vi "Measurement Logic.vi"() -> ()   [LabVIEW 2021, in "Eff And Load Reg_Channel Ganging.lvlib"]
uses:
  Eff And Load Reg_Channel Ganging.lvlib
  Measurement Configuration.ctl
  Measurement Results.ctl
  <vilib>/Plug-In SDKs/Measurements/Measure Call Context/Measure Call Context.lvclass
  shared/Ganging/controls/Power ON-Ganging.ctl
  shared/Single/controls/Power ON-Single.ctl
panel:
  out "measure call context out":refnum<class "Measure Call Context.lvclass">
  in  "measure call context in":refnum<class "Measure Call Context.lvclass">
  out "measurement results":T1
  in  "measurement configuration":T2={"Mode of operation"=enum."Power on the DUT", "Source resource names"=[], "Load resource names"=[], "Power ON output function"=1006, "Power ON/Source system configuration"=enum."Parallel", "Power ON V/I Source start level"=6.0, "Source stop voltage"=14.0, "Source voltage sweep points"=4, "Source voltage level range"=20.0, "Power ON/Source sense"=1009, "Source limit symmetry"=enum."Asymmetric", "Power ON/Source current/voltage limit range"=25.0, "Source current limit low"=-0.6, "Source current limit high"=25.0, "Source transient response"=1038, "Source voltage gain bandwidth"=2000.0, "Source voltage compensation frequency"=3530.0, "Source voltage pole-zero ratio"=2.0, "Load system configuration"=enum."Parallel", "Load device voltage/current rating"=50.0, "Load start current"=1.0, "Load stop current"=50.0, "Load current sweep points/points per decade"=10, "Load sweep type"="Logarithmic", "Load current level range"=80.0, "Load sense"=1009, "Load limit symmetry"=enum."Symmetric", "Load voltage limit range"=6.0, "Load voltage limit low"=0.0, "Load voltage limit high"=inf, "Load transient response"=1038, "Load current gain bandwidth"=14000.0, "Load current compensation frequency"=180000.0, "Load current pole-zero ratio"=0.3, "DUT setup time"=1.0, "Source delay"=0.005, "Aperture time"=0.005, "Nominal output voltage"=1.0, "Measurement timeout"=10.0} {"Power ON output function" items=["Series", "Parallel", "Manual"]; "Nominal output voltage" format="%#_6pA"; "Source voltage sweep points" format="%#_6p"; "Power ON V/I Source start level" format="%#_6p"; "Load sense" items=["Symmetric", "Asymmetric"]; "Load transient response" items=["Slow"=1041, "Normal"=1038, "Fast"=1039, "Custom"=1042]; "Power ON/Source sense" items=["Symmetric", "Asymmetric"]; "Source transient response" items=["Slow"=1041, "Normal"=1038, "Fast"=1039, "Custom"=1042]; "Load voltage limit high" format="%#_6p"; "Load voltage limit low" format="%#_6p"; "Load voltage limit range" format="%#_6p"; "Load current level range" format="%#_6p"; "Source current limit high" format="%#_6p"; "Source current limit low" format="%#_6p"; "Power ON/Source current/voltage limit range" format="%#_6p"; "Source voltage level range" format="%#_6p"}
  out "error out":errorcluster
  in  "error in":errorcluster
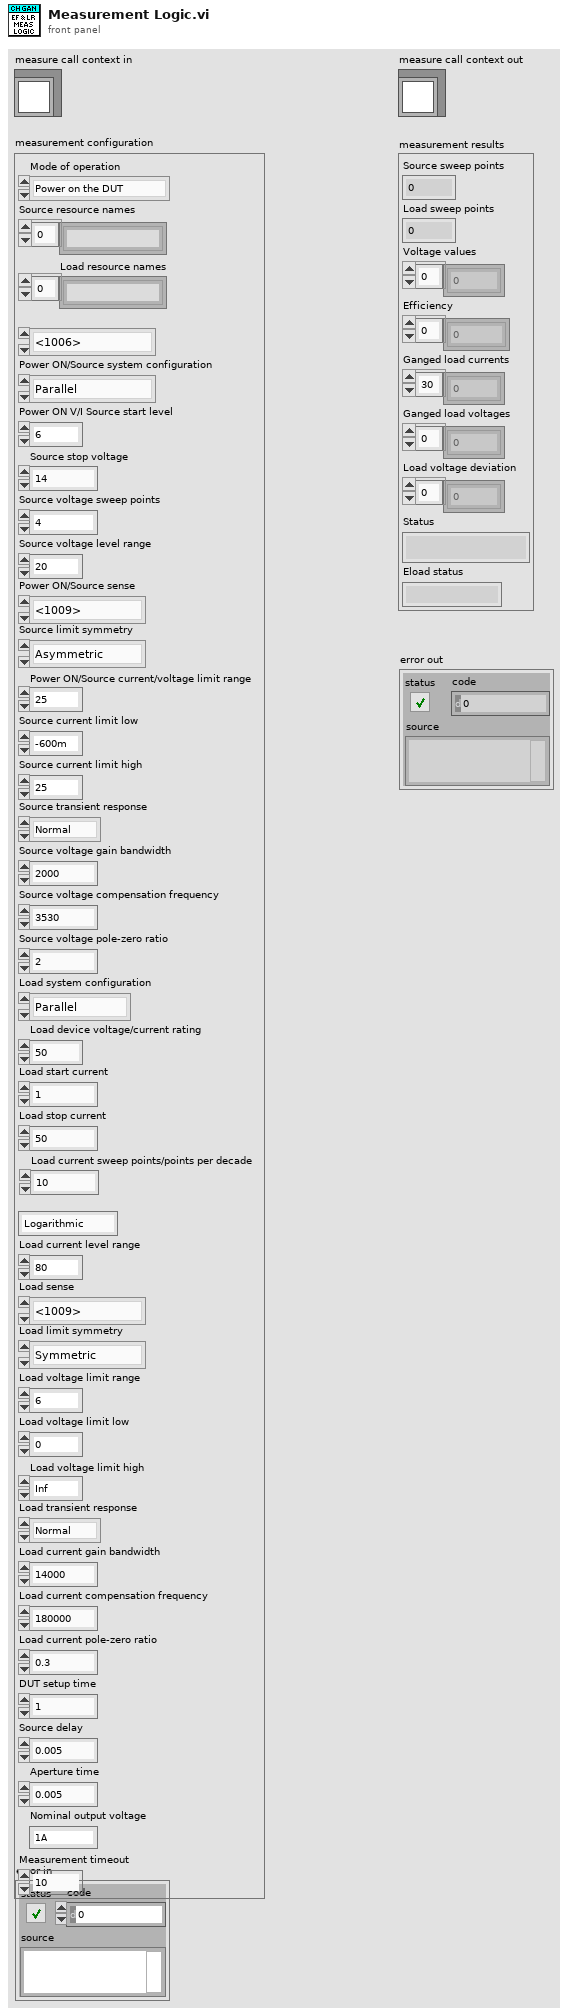
[diagram p1: front panel]
types:
  T1 = typedef "Eff And Load Reg_Channel Ganging.lvlib/Measurement Results.ctl" = cluster{"Source sweep points":i32, "Load sweep points":i32, "Voltage values":dbl[], "Efficiency":dbl[], "Ganged load currents":dbl[], "Ganged load voltages":dbl[], "Load voltage deviation":dbl[], "Status":string, "Eload status":string}
  T2 = typedef "Eff And Load Reg_Channel Ganging.lvlib/Measurement Configuration.ctl" = cluster{"Mode of operation":enum32{"Power on the DUT", "Perform measurement", "Power off the DUT"}, "Source resource names":string[], "Load resource names":string[], "Power ON output function":i32, "Power ON/Source system configuration":enum32{"Series", "Parallel", "Manual"}, "Power ON V/I Source start level":dbl, "Source stop voltage":dbl, "Source voltage sweep points":i32, "Source voltage level range":dbl, "Power ON/Source sense":i32, "Source limit symmetry":enum32{"Symmetric", "Asymmetric"}, "Power ON/Source current/voltage limit range":dbl, "Source current limit low":dbl, "Source current limit high":dbl, "Source transient response":i32, "Source voltage gain bandwidth":dbl, "Source voltage compensation frequency":dbl, "Source voltage pole-zero ratio":dbl, "Load system configuration":enum32{"Series", "Parallel", "Manual"}, "Load device voltage/current rating":dbl, "Load start current":dbl, "Load stop current":dbl, "Load current sweep points/points per decade":i32, "Load sweep type":string, "Load current level range":dbl, "Load sense":i32, "Load limit symmetry":enum32{"Symmetric", "Asymmetric"}, "Load voltage limit range":dbl, "Load voltage limit low":dbl, "Load voltage limit high":dbl, "Load transient response":i32, "Load current gain bandwidth":dbl, "Load current compensation frequency":dbl, "Load current pole-zero ratio":dbl, "DUT setup time":dbl, "Source delay":dbl, "Aperture time":dbl, "Nominal output voltage":dbl, "Measurement timeout":dbl}
  T3 = enum32{"Power on the DUT", "Perform measurement", "Power off the DUT"}
  T4 = typedef "Power ON-Ganging.ctl" = cluster{"Master/single Resource name":string, "Slave resource name":string[], "System configuration":enum32{"Series", "Parallel", "Manual"}, "Output function":i32, "Voltage/current level":dbl, "Voltage/current limit":dbl, "Sense":i32}
  T5 = typedef "Power ON-Single.ctl" = cluster{"Voltage/current level":dbl, "Voltage/current limit":dbl, "Sense":i32, "Resource name":string, "Output function":i32}
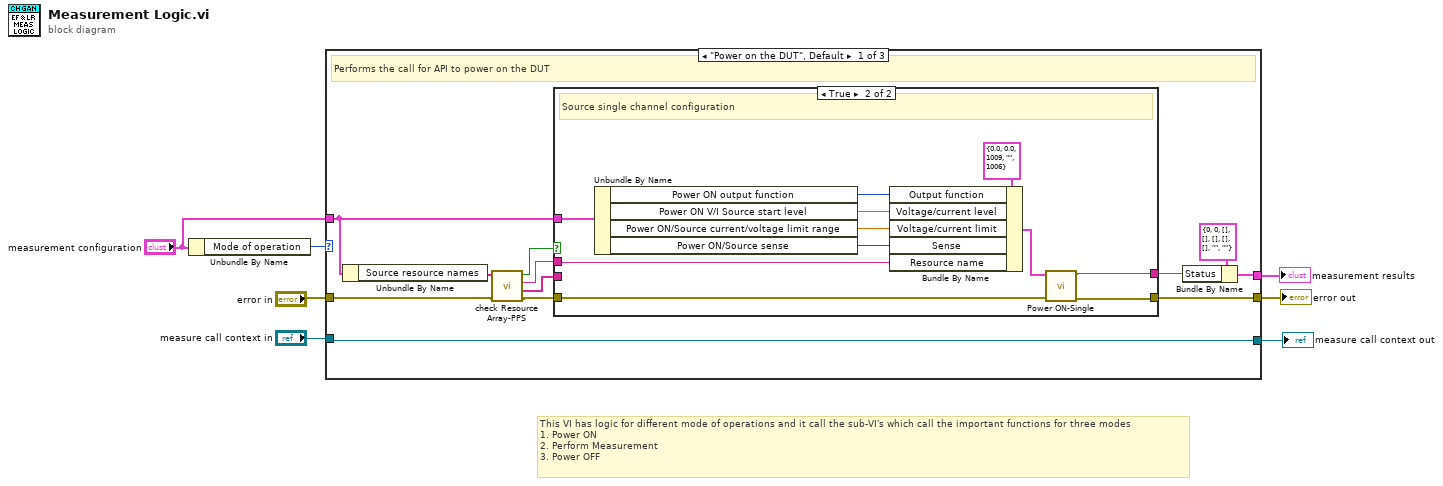
[diagram p0: block diagram]
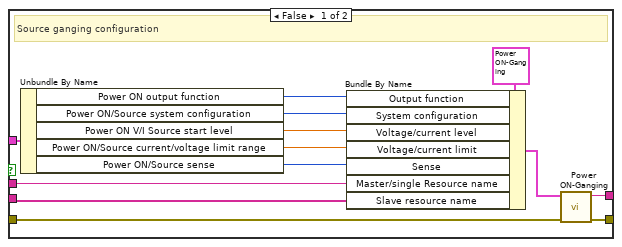
[diagram p2: hidden frame]
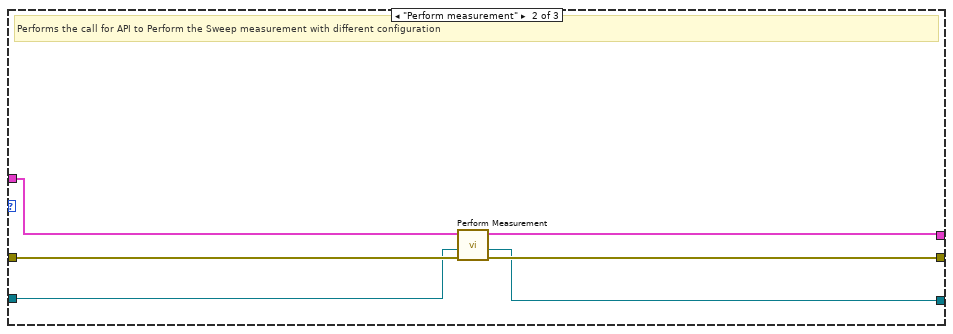
[diagram p3: hidden frame]
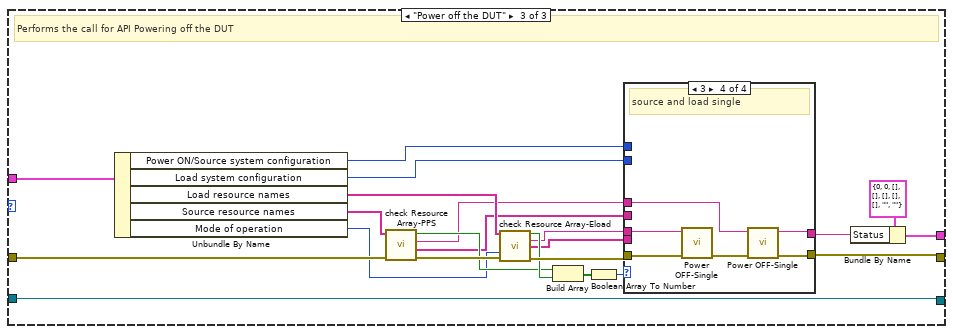
[diagram p4: hidden frame]
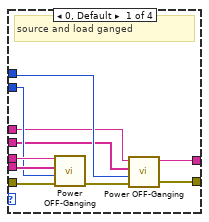
[diagram p5: hidden frame]
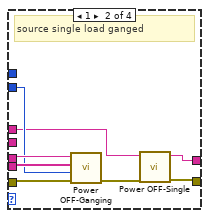
[diagram p6: hidden frame]
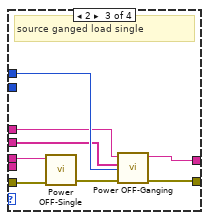
[diagram p7: hidden frame]
diagram:
  # "This VI has logic for different mode of operations and it call the sub-VI's which call the important functions for three modes\n1. Power ON\n2. Perform Measurement\n3. Power OFF"
  n1 = Unbundle By Name("measurement configuration") -> ("Mode of operation"=w7:T3)
  n2 = case shown="\"Power on the DUT\", Default" w7 {
    tunnel: "measurement configuration" -> [w14 w45 w57]
    tunnel: "error in" -> [w13 w49 w56]
    tunnel: [w12 w48 w55] -> w5
    tunnel: [w11 w47 w53] -> w3
    tunnel: "measure call context in" -> [w11 w46 w53]
    tunnel: [w8 w44 w51] -> w1
    frame "Power on the DUT", Default {
      # "Performs the call for API to power on the DUT"
      n3 = Unbundle By Name(w14) -> ("Source resource names"=w16:string[])
      n4 = call "check Resource Array-PPS.vi"("error in"=w13, "Resource names"=w16) -> ("error out"=w19:errorcluster, "Slave resource names"=w17:string[], "Single/Master resouce names"=w18:string, "Single or ganged configuration"=w15:bool)  [unwired: 6 in]
      n5 = case shown="True" w15 {
        tunnel: w19 -> [w27 w42]
        tunnel: [w28 w41] -> w12
        tunnel: w17 -> [w30 _]
        tunnel: w14 -> [w32 w43]
        tunnel: w18 -> [w31 w38]
        tunnel: [w29 w40] -> w10
        frame False {
          # "Source ganging configuration"
          n6 = Unbundle By Name(w32) -> ("Power ON output function"=w20:i32, "Power ON/Source system configuration"=w24:enum32{"Series", "Parallel", "Manual"}, "Power ON V/I Source start level"=w23:dbl, "Power ON/Source current/voltage limit range"=w22:dbl, "Power ON/Source sense"=w21:i32)
          n7 = Bundle By Name(cluster=T4 {"Master/single Resource name"="", "Slave resource name"=[], "System configuration"=enum."Parallel", "Output function"=1006, "Voltage/current level"=0.0, "Voltage/current limit"=0.0, "Sense"=1009} ("Power ON"), "Output function"=w20, "System configuration"=w24, "Voltage/current level"=w23, "Voltage/current limit"=w22, "Sense"=w21, "Master/single Resource name"=w31, "Slave resource name"=w30) -> (w25:T4)
          n8 = call "Power ON-Ganging.vi"("error in"=w27, "Power ON"=w25) -> ("error out"=w28:errorcluster, "Status"=w29:string)  [unwired: 8 in]
        }
        frame True {
          # "Source single channel configuration"
          n9 = Unbundle By Name(w43) -> ("Power ON output function"=w33:i32, "Power ON V/I Source start level"=w36:dbl, "Power ON/Source current/voltage limit range"=w35:dbl, "Power ON/Source sense"=w34:i32)
          n10 = Bundle By Name(cluster=T5 {"Voltage/current level"=0.0, "Voltage/current limit"=0.0, "Sense"=1009, "Resource name"="", "Output function"=1006} ("Power ON single"), "Output function"=w33, "Voltage/current level"=w36, "Voltage/current limit"=w35, "Sense"=w34, "Resource name"=w38) -> (w39:T5)
          n11 = call "Power ON-Single.vi"("error in"=w42, "Power ON single"=w39) -> ("error out"=w41:errorcluster, "Status"=w40:string)  [unwired: 8 in]
        }
      }
      n12 = Bundle By Name(cluster=T1 {"Source sweep points"=0, "Load sweep points"=0, "Voltage values"=[], "Efficiency"=[], "Ganged load currents"=[], "Ganged load voltages"=[], "Load voltage deviation"=[], "Status"="", "Eload status"=""} ("measurement results"), "Status"=w10) -> (w8:T1)
    }
    frame "Perform measurement" {
      # "Performs the call for API to Perform the Sweep measurement with different configuration"
      n13 = call "Perform Measurement.vi"("error in"=w49, "Measure Call Context in"=w46, "measurement configuration"=w45) -> ("error out"=w48:errorcluster, "Measure Call Context out"=w47:refnum<class "Measure Call Context.lvclass">, "measurement results"=w44:T1)  [unwired: 5 in]
    }
    frame "Power off the DUT" {
      # "Performs the call for API Powering off the DUT"
      n14 = Unbundle By Name(w57) -> ("Power ON/Source system configuration"=w68:enum32{"Series", "Parallel", "Manual"}, "Load system configuration"=w69:enum32{"Series", "Parallel", "Manual"}, "Load resource names"=w63:string[], "Source resource names"=w61:string[], "Mode of operation"=w50:T3)
      n15 = call "check Resource Array-PPS.vi"("error in"=w56, "Resource names"=w61) -> ("error out"=w62:errorcluster, "Slave resource names"=w58:string[], "Single/Master resouce names"=w59:string, "Single or ganged configuration"=w60:bool)  [unwired: 6 in]
      n16 = call "check Resource Array-Eload.vi"("Resource names"=w63, "Mode of operation"=w50, "error in"=w62) -> ("Single or ganged configuration"=w66:bool, "Single/Master resouce name"=w65:string, "Slave resource names"=w64:string[], "error out"=w67:errorcluster)  [unwired: 8 in, 1 out]
      n17 = Build Array(w60, w66) -> (w71:bool[])
      n18 = Boolean Array To Number(Boolean array=w71) -> (number=w70:u32)
      n19 = case shown="3" w70 {
        tunnel: w67 -> [w80 w89 w97 w103]
        tunnel: [w72 w87 w90 w101] -> w55
        tunnel: [w81 w88 w93 w99] -> w54
        tunnel: w65 -> [w79 w86 w96 w100]
        tunnel: w64 -> [w78 w85 _ _]
        tunnel: w69 -> [w77 w84 _ _]
        tunnel: w68 -> [w76 _ w94 _]
        tunnel: w59 -> [w74 w83 w92 w98]
        tunnel: w58 -> [w75 _ w91 _]
        frame 0, Default {
          # "source and load ganged"
          n20 = call "Power OFF-Ganging.vi"("error in"=w80, "Ganged Config"=w77, "Slave resource names"=w78, "Master resouce name"=w79) -> ("error out"=w73:errorcluster)  [unwired: 6 in, 1 out]
          n21 = call "Power OFF-Ganging.vi"("error in"=w73, "Ganged Config"=w76, "Slave resource names"=w75, "Master resouce name"=w74) -> ("error out"=w72:errorcluster, "Status"=w81:string)  [unwired: 6 in]
        }
        frame 1 {
          # "source single load ganged"
          n22 = call "Power OFF-Ganging.vi"("error in"=w89, "Ganged Config"=w84, "Slave resource names"=w85, "Master resouce name"=w86) -> ("error out"=w82:errorcluster)  [unwired: 6 in, 1 out]
          n23 = call "Power OFF-Single.vi"("error in (no error)"=w82, "Resource name"=w83) -> ("error out"=w87:errorcluster, "Status"=w88:string)  [unwired: 8 in]
        }
        frame 2 {
          # "source ganged load single"
          n24 = call "Power OFF-Single.vi"("error in (no error)"=w97, "Resource name"=w96) -> ("error out"=w95:errorcluster)  [unwired: 8 in, 1 out]
          n25 = call "Power OFF-Ganging.vi"("error in"=w95, "Ganged Config"=w94, "Slave resource names"=w91, "Master resouce name"=w92) -> ("error out"=w90:errorcluster, "Status"=w93:string)  [unwired: 6 in]
        }
        frame 3 {
          # "source and load single"
          n26 = call "Power OFF-Single.vi"("error in (no error)"=w103, "Resource name"=w100) -> ("error out"=w102:errorcluster)  [unwired: 8 in, 1 out]
          n27 = call "Power OFF-Single.vi"("error in (no error)"=w102, "Resource name"=w98) -> ("error out"=w101:errorcluster, "Status"=w99:string)  [unwired: 8 in]
        }
      }
      n28 = Bundle By Name(cluster=T1 {"Source sweep points"=0, "Load sweep points"=0, "Voltage values"=[], "Efficiency"=[], "Ganged load currents"=[], "Ganged load voltages"=[], "Load voltage deviation"=[], "Status"="", "Eload status"=""} ("measurement results"), "Status"=w54) -> (w51:T1)
    }
  }
  "error out" <- w5
  "measurement results" <- w1
  "measure call context out" <- w3
